vi "build-diode-scan-pts.vi"(6 "Y step size":dbl, 7 "X step size":dbl=0.5 format="%#_13g", 8 "Y end":dbl=121.5 format="%#_13g", 9 "Y start":dbl=120.5 format="%#_13g", 10 "X end":i32=263, 11 "X start":i32=262) -> (2 "y":dbl[](array[numeric]), 3 "x":dbl[](array[numeric]))   [LabVIEW 2024]
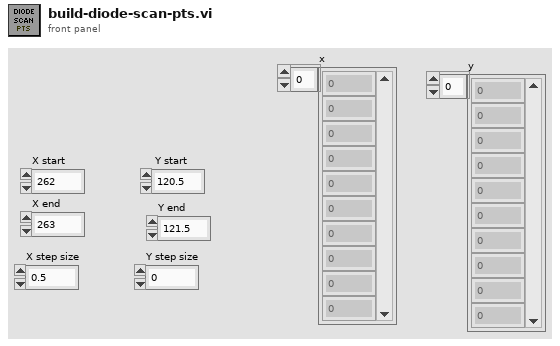
[diagram p1: front panel]
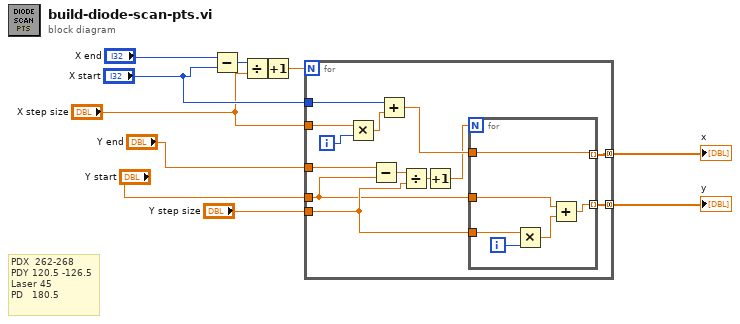
[diagram p0: block diagram]
diagram:
  # "PDX  262-268\nPDY 120.5 -126.5\nLaser 45\nPD   180.5"
  n1 = Subtract(x="X end", y="X start") -> (x-y=w11:i32)
  n2 = Divide(x=w11, y="X step size") -> (x/y=w9:dbl)
  n3 = Increment(x=w9) -> (x+1=w7:dbl)
  n4 = for {
    N: w7 -> [_]
    tunnel: "X start" -> [w23]
    tunnel: [w20] -> w6 mode=concatenating
    tunnel: [w19] -> w5 mode=concatenating
    tunnel: "X step size" -> [w15]
    tunnel: "Y step size" -> [w14]
    tunnel: "Y end" -> [w13]
    tunnel: "Y start" -> [w12]
    i -> [w24]
    n5 = Multiply(x=w15, y=w24) -> (x*y=w22:dbl)
    n6 = Subtract(x=w13, y=w12) -> (x-y=w18:dbl)
    n7 = Add(x=w23, y=w22) -> (x+y=w21:dbl)
    n8 = Divide(x=w18, y=w14) -> (x/y=w17:dbl)
    n9 = Increment(x=w17) -> (x+1=w16:dbl)
    n10 = for {
      N: w16 -> [_]
      tunnel: w21 -> [w30]
      tunnel: [w30] -> w20 mode=indexing
      tunnel: [w27] -> w19 mode=indexing
      tunnel: w14 -> [w26]
      tunnel: w12 -> [w25]
      i -> [w28]
      n11 = Multiply(x=w26, y=w28) -> (x*y=w29:dbl)
      n12 = Add(x=w25, y=w29) -> (x+y=w27:dbl)
    }
  }
  "x" <- w6
  "y" <- w5
